vi "Interpolate 2D Scattered_Linear.vi"(0 "X":dbl[](array[numeric]), 5 "Y":dbl[](array[numeric]), 7 "Z":dbl[](array[numeric]), 9 "Xi":dbl[](array[numeric]), 11 "Yi":dbl[](array[numeric])) -> (4 "Zi":dbl[](array[numeric]), 15 "error":i32)   [LabVIEW 2020, in "NI_AAL_Interpolation.lvlib"]
uses:
  <vilib>/gmath/NI_AAL_Interpolation.lvlib
  <vilib>/Analysis/NI_AAL_Geometry.lvlib
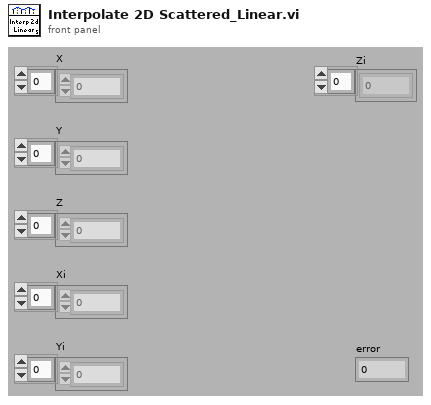
[diagram p1: front panel]
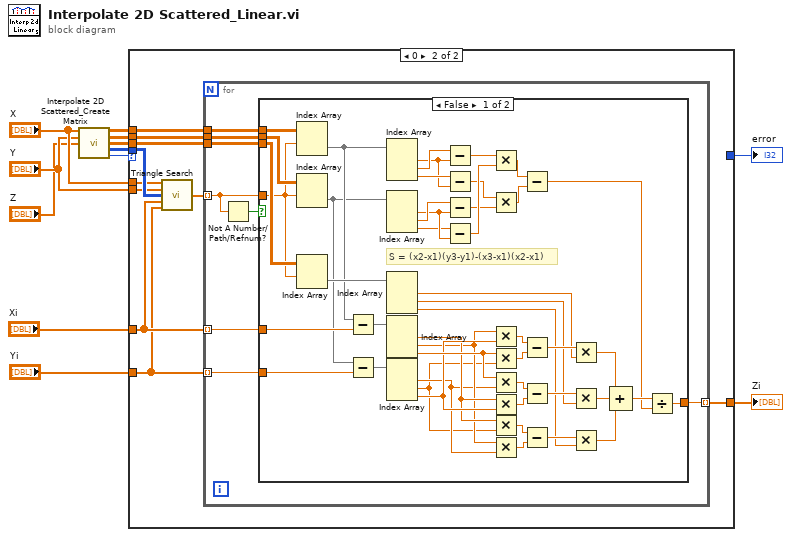
[diagram p0: block diagram]
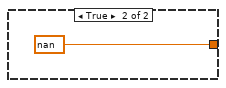
[diagram p3: hidden frame]
diagram:
  n1 = call <vilib>:"Interpolate 2D Scattered_Create Matrix.vi"("X"="X", "Y"="Y", "Z"="Z") -> ("X(Tri)"=w3:dbl[][], "Y(Tri)"=w2:dbl[][], "Z(Tri)"=w1:dbl[][], "Triangles"=w10:i32[][], "error"=w6:i32)  [unwired: 8 out]
  n2 = case shown="0" w6 {
    selector: w6 -> [w13 _]
    tunnel: "Xi" -> [_ w22]
    tunnel: "Yi" -> [_ w21]
    tunnel: w10 -> [_ w20]
    tunnel: "X" -> [_ w19]
    tunnel: "Y" -> [_ w18]
    tunnel: [_ w17] -> w7
    tunnel: [w13 _] -> w5
    tunnel: w3 -> [_ w16]
    tunnel: w2 -> [_ w15]
    tunnel: w1 -> [_ w14]
    frame -1, Default {
    }
    frame 0 {
      n3 = call <vilib>:"Triangle Search.vi"("X"=w19, "Y"=w18, "Triangles"=w20, "Xi"=w22, "Yi"=w21) -> ("indices"=w23:dbl[])  [unwired: 10 out]
      n4 = for {
        tunnel: w23 -> [w30] mode=indexing
        tunnel: w22 -> [w29] mode=indexing
        tunnel: w21 -> [w28] mode=indexing
        tunnel: [w27] -> w17 mode=indexing
        tunnel: w16 -> [w26]
        tunnel: w15 -> [w25]
        tunnel: w14 -> [w24]
        n5 = Not A Number/Path/Refnum?(number/path/refnum=w30) -> (NaN/Path/Refnum?=w31:bool)
        n6 = case shown="False" w31 {
          tunnel: w30 -> [w34 _]
          tunnel: w29 -> [w78 _]
          tunnel: w28 -> [w77 _]
          tunnel: [w40 nan] -> w27
          tunnel: w26 -> [w38 _]
          tunnel: w25 -> [w37 _]
          tunnel: w24 -> [w35 _]
          frame False {
            # "S = (x2-x1)(y3-y1)-(x3-x1)(x2-x1)"
            n7 = Index Array(array=w38, index (row)=w34) -> (element=w33:dbl[])  [unwired: 1 in]
            n8 = Index Array(array=w37, index (row)=w34) -> (element=w32:dbl[])  [unwired: 1 in]
            n9 = Index Array(array=w35, index (row)=w34) -> (element=w36:dbl[])  [unwired: 1 in]
            n10 = Subtract(x=w33, y=w78) -> (x-y=w76:dbl[])
            n11 = Subtract(x=w32, y=w77) -> (x-y=w75:dbl[])
            n12 = Index Array(array=w33) -> (element #1=w51:dbl, element #2=w54:dbl, element #3=w53:dbl)  [unwired: 3 in]
            n13 = Index Array(array=w32) -> (element #1=w50:dbl, element #2=w52:dbl, element #3=w49:dbl)  [unwired: 3 in]
            n14 = Index Array(array=w36) -> (element #1=w62:dbl, element #2=w60:dbl, element #3=w58:dbl)  [unwired: 3 in]
            n15 = Index Array(array=w76) -> (element #1=w72:dbl, element #2=w71:dbl, element #3=w74:dbl)  [unwired: 3 in]
            n16 = Index Array(array=w75) -> (element #1=w70:dbl, element #2=w39:dbl, element #3=w73:dbl)  [unwired: 3 in]
            n17 = Subtract(x=w54, y=w51) -> (x-y=w48:dbl)
            n18 = Subtract(x=w53, y=w51) -> (x-y=w45:dbl)
            n19 = Subtract(x=w52, y=w50) -> (x-y=w46:dbl)
            n20 = Subtract(x=w49, y=w50) -> (x-y=w47:dbl)
            n21 = Multiply(x=w48, y=w47) -> (x*y=w44:dbl)
            n22 = Multiply(x=w45, y=w46) -> (x*y=w43:dbl)
            n23 = Multiply(x=w71, y=w73) -> (x*y=w68:dbl)
            n24 = Multiply(x=w74, y=w39) -> (x*y=w69:dbl)
            n25 = Multiply(x=w74, y=w70) -> (x*y=w67:dbl)
            n26 = Multiply(x=w72, y=w73) -> (x*y=w66:dbl)
            n27 = Multiply(x=w72, y=w39) -> (x*y=w65:dbl)
            n28 = Multiply(x=w71, y=w70) -> (x*y=w64:dbl)
            n29 = Subtract(x=w44, y=w43) -> (x-y=w41:dbl)
            n30 = Subtract(x=w68, y=w69) -> (x-y=w63:dbl)
            n31 = Subtract(x=w67, y=w66) -> (x-y=w61:dbl)
            n32 = Subtract(x=w65, y=w64) -> (x-y=w59:dbl)
            n33 = Multiply(x=w63, y=w62) -> (x*y=w57:dbl)
            n34 = Multiply(x=w61, y=w60) -> (x*y=w56:dbl)
            n35 = Multiply(x=w59, y=w58) -> (x*y=w55:dbl)
            n36 = Compound Arithmetic op=ADD(w57, w56, w55) -> (w42:dbl)
            n37 = Divide(x=w42, y=w41) -> (x/y=w40:dbl)
          }
          frame True {
          }
        }
      }
    }
  }
  "Zi" <- w7
  "error" <- w5
